vi "GetParam.vi"(8 "error in (no error)":errorcluster caption="entrée d'erreur (pas d'erreur)", 11 "Sparse_Uncorrelated.lvclass":refnum<class "Sparse_Uncorrelated.lvclass">) -> (0 "error out":errorcluster caption="sortie d'erreur", 2 "make_sparse_uncorrelated":T1={"n_samples"=100, "n_features"=10, "random_state"=-1, "Returns"="X"} {"random_state" min=-1; "n_samples" min=1}, 3 "Sparse_Uncorrelated.lvclass":refnum<class "Sparse_Uncorrelated.lvclass">)   [LabVIEW 2020, in "Sparse_Uncorrelated.lvclass"]
doc: "Get Parameters"
uses:
  Sparse_Uncorrelated.lvclass
  Sparse_Uncorrelated.lvclass/Sparse_Uncorrelated.ctl
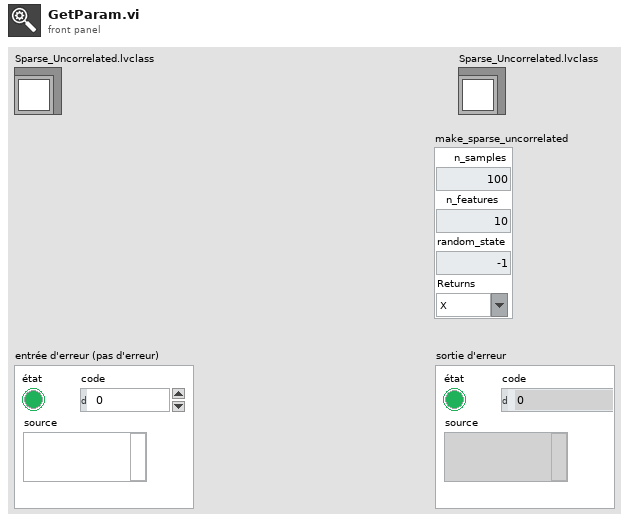
[diagram p1: front panel]
types:
  T1 = cluster{"n_samples":u32, "n_features":i32, "random_state":i32, "Returns":string}
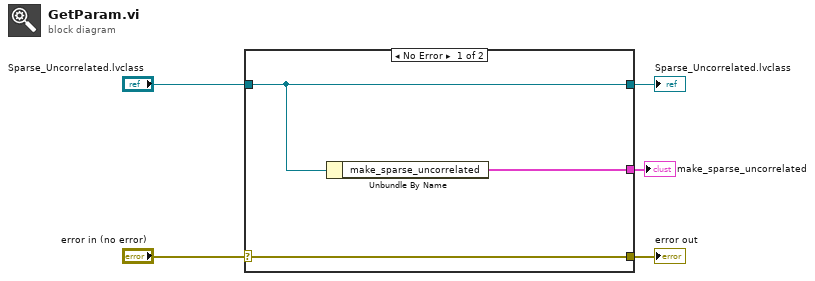
[diagram p0: block diagram]
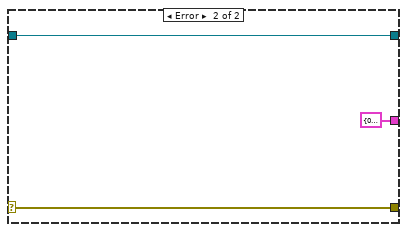
[diagram p2: hidden frame]
diagram:
  n1 = case shown="No Error" "error in (no error)" {
    selector: "error in (no error)" -> [w8 w10]
    tunnel: [w8 w10] -> w4
    tunnel: [w7 w11] -> w2
    tunnel: "Sparse_Uncorrelated.lvclass" -> [w7 w11]
    tunnel: [w6 T1 {"n_samples"=0, "n_features"=0, "random_state"=0, "Returns"=""} ("make_sparse_uncorrelated")] -> w1
    frame No Error {
      n2 = Unbundle By Name(w7) -> ("make_sparse_uncorrelated"=w6:T1)
    }
    frame Error {
    }
  }
  "error out" <- w4
  "Sparse_Uncorrelated.lvclass" <- w2
  "make_sparse_uncorrelated" <- w1
